vi "Set Trigger Data.vi"(10 "Trigger Data":string, 11 "Assembler in":refnum<class "Assembler.lvclass">) -> (3 "Assembler out":refnum<class "Assembler.lvclass">)   [LabVIEW 2019, in "TimingDRV Engine.lvlib" / "Assembler.lvclass"]
uses:
  Assembler.lvclass
  Assembler.lvclass/Assembler.ctl
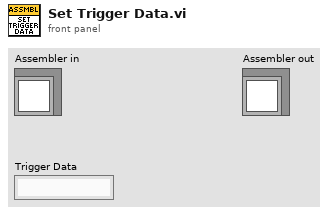
[diagram p1: front panel]
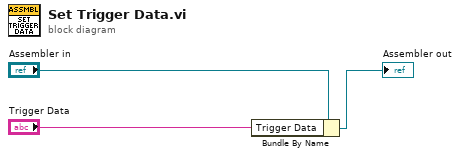
[diagram p0: block diagram]
diagram:
  n1 = Bundle By Name(cluster="Assembler in", "Trigger Data"="Trigger Data") -> (→"Assembler out":refnum<class "Assembler.lvclass">)
